vi "Read Data Available.vi"(8 "error in":errorcluster, 11 "GUI In":refnum<class "GUI.lvclass">) -> (0 "error out":errorcluster, 2 "Data Available":refnum<notifier>, 3 "GUI Out":refnum<class "GUI.lvclass">)   [LabVIEW 2012, in "GUI.lvclass"]
uses:
  Reusable/GUI/GUI.lvclass
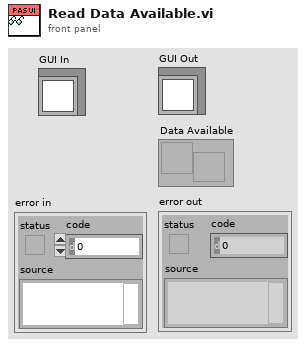
[diagram p1: front panel]
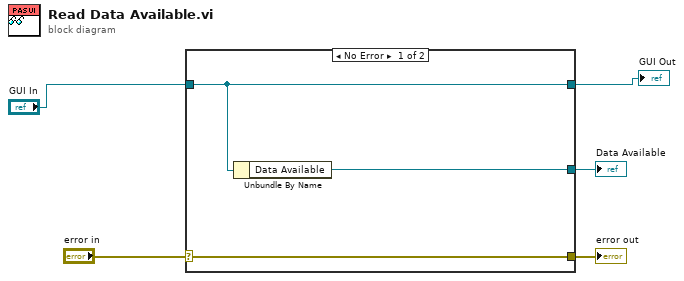
[diagram p0: block diagram]
diagram:
  n1 = case shown="No Error" "error in" {
    selector: "error in" -> [w8 w9]
    tunnel: [w8 w9] -> w4
    tunnel: [w7 w10] -> w1
    tunnel: "GUI In" -> [w7 w10]
    tunnel: [w6 _] -> w3
    frame No Error {
      n2 = Unbundle By Name(w7) -> ("Data Available"=w6:refnum<notifier>)
    }
    frame Error {
    }
  }
  "error out" <- w4
  "Data Available" <- w3
  "GUI Out" <- w1
